vi "Target Analyze.vi"(0 "Original Image_in":T1, 1 "Target Choice":i8(knob) scale=0.0..2.0, 5 "Color Plane":i32(ring) items=["Red", "Green", "Blue", "Hue", "Saturation", "Luminance", "Value", "Intensity"], 7 "Range":cluster{"Lower value":sgl, "Upper value":sgl}={"Lower value"=150.0, "Upper value"=255.0} {"Lower value" scale=0.0..255.0; "Upper value" scale=0.0..255.0}, 9 "Camera Type":enum16{"206", "1011"}(ring)=enum."1011", 11 "Annotate":bool=TRUE) -> (3 "Target Info":T2(array[cluster]), 4 "Original Image_out":T1(plugin-control), 6 "Processed Image":T1(plugin-control), 8 "Distance [m]":dbl, 10 "Position of Target Center X":dbl, 14 "Center Target":bool, 15 "Position of Target Center Y":dbl)   [LabVIEW 2012]
doc: "This VI demonstrates how to do target processing on a laptop computer. It uses the same MJPG VI as the dashboard, sets a few of the important camera properties that impact processing, and carries out the same processing steps as the RT example also included in this project."
uses:
  <vilib>/vision/Image Controls.llb/IMAQ Image.ctl
  <vilib>/vision/NI_Vision_Development_Module.lvlib
panel:
  out "Target":bool
  out "Numeric Target Info (X,Y,D)":dbl[](array[numeric])
  in  "Area Size Limit %":dbl=0.5
  in  "Particle Count Limit":i32=10
  in  "Score Limits":T3={"Rect Coverage"=60.0, "X Edge Strength"=40.0, "Y Edge Strength"=60.0, "Center"=75.0, "Outer"=75.0}
  in  "Processing":enum32{"Monochrome", "Color"}(tab)
  out "Value 2":cluster{i32, i32}
  out "Saturation 2":cluster{i32, i32}
  in  "Value":i32=255
  in  "Saturation":i32=255
  in  "Hue 2":i32(knob)=65 scale=0.0..255.0
  in  "Margins":cluster{"Hue":i32, "Sat":i32, "Val":i32}={"Hue"=33, "Sat"=53, "Val"=9} {"Sat" scale=0.0..80.0; "Val" scale=0.0..80.0; "Hue" scale=0.0..80.0}
  out "Hue":cluster{i32, i32}
  # "Information:\nProcessing can be based on color or light intensity.\nParticles within the image are scored by rectangle coverage, aspect ratio, and\nedge strength/hollowness. A particle is considered a target if all scores\nare above the score limits you set. Particles can be annotated -- surrounded by\na rectangle and scores drawn to the left .\nTo control the number of particles being scored, use the count limit and the size\nlimit.\nBe sure to set the Camera IP before running. The distance calculation uses the\ncamera type to index the value of the lens view angle."
  # "Click in the image to choose  color for processing."
  # "Green scores are above the limit, orange are below. Inner/outer rect\nindicates all passed."
  # "Lower/Upper"
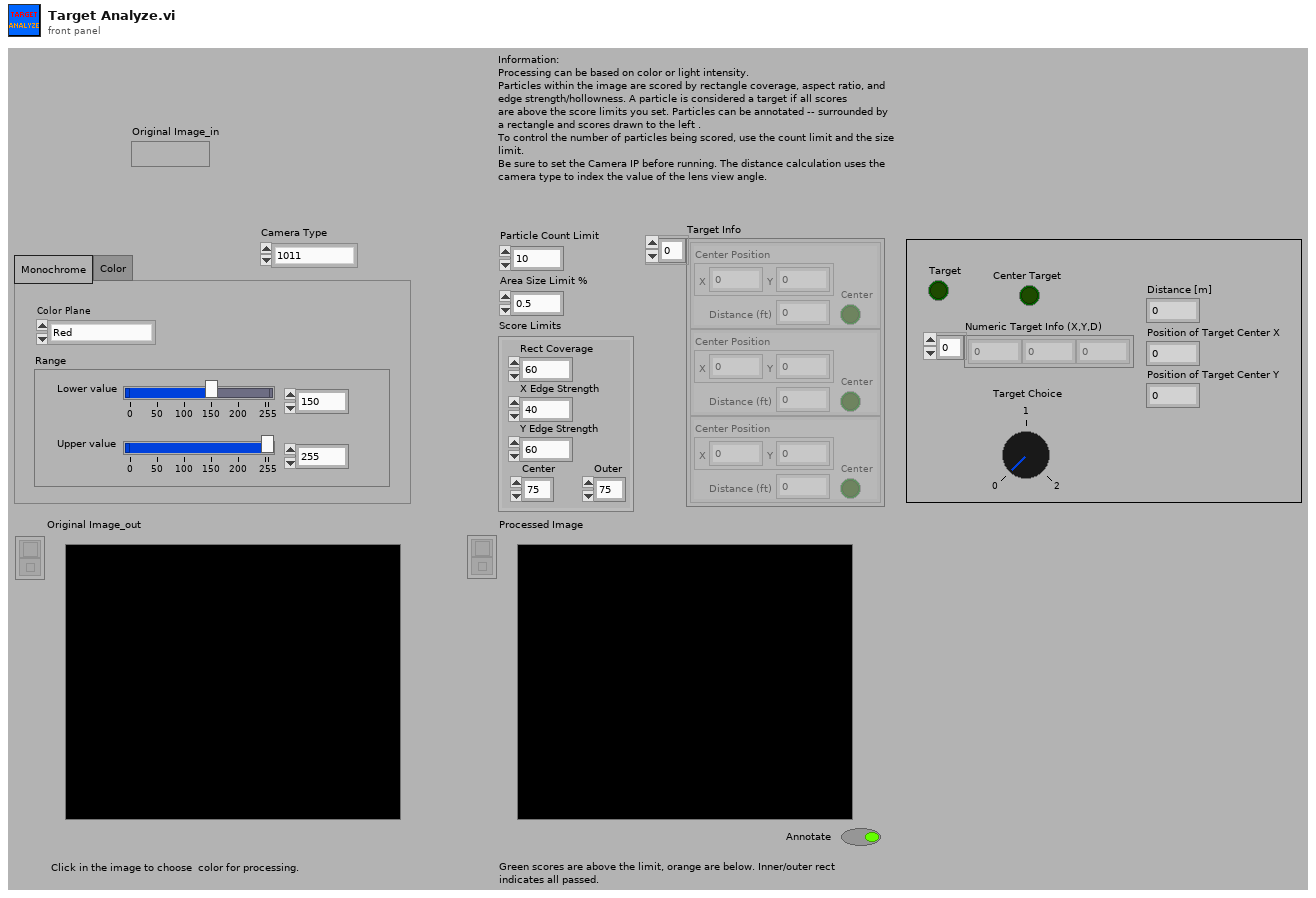
[diagram p1: front panel]
types:
  T1 = typedef "IMAQ Image.ctl" = refnum<image>
  T2 = cluster{"Center Position":cluster{"X":dbl, "Y":dbl}, "Distance (ft)":dbl, "Center":bool}[]
  T3 = cluster{"Rect Coverage":dbl, "X Edge Strength":dbl, "Y Edge Strength":dbl, "Center":dbl, "Outer":dbl}
  T4 = cluster{"Position":cluster{"X":dbl, "Y":dbl}, "Distance (ft)":dbl, "Center Target":bool}[]
  T5 = typedef "Image Type" = u32
  T6 = cluster{cluster{"Left":dbl, "Top":dbl, "Right":dbl, "Bottom":dbl}, "Scores":dbl[], cluster{"Long":dbl, "Short":dbl}}[]
  T7 = cluster{"Target Center (-1 to 1)":cluster{"X":dbl, "Y":dbl}, "Distance (ft)":dbl, "Center Target":bool}
  T8 = cluster{"Target Center (-1 to 1)":cluster{"X":dbl, "Y":dbl}, "Distance (ft)":dbl, "Center Target":bool}[]
  T9 = cluster{"Position":cluster{"X":dbl, "Y":dbl}, "Distance (ft)":dbl, "Center Target":bool}
  T10 = cluster{"Left":dbl, "Top":dbl, "Right":dbl, "Bottom":dbl}
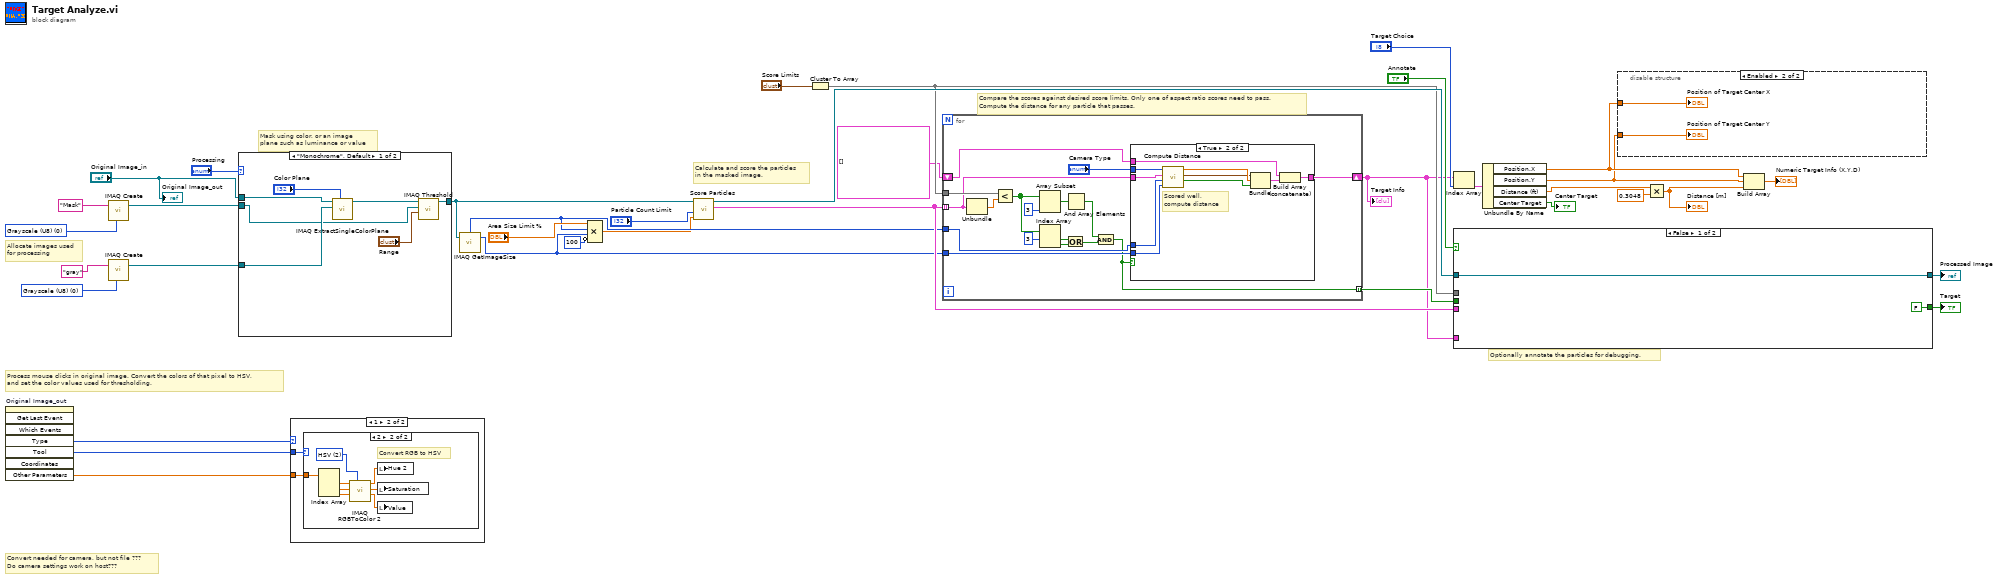
[diagram p0: block diagram]
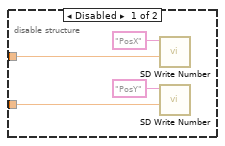
[diagram p2: hidden frame]
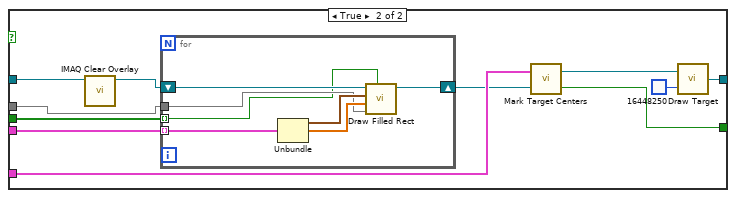
[diagram p3: hidden frame]
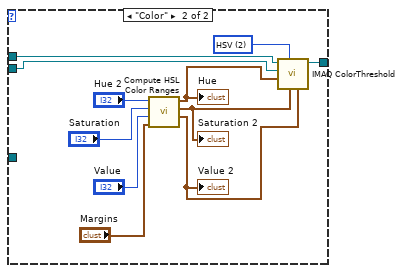
[diagram p4: hidden frame]
diagram:
  w33 = T5 0 items=["Grayscale (U8)", "Grayscale (I16)", "Grayscale (SGL)", "Complex (CSG)", "RGB (U32)", "HSL (U32)", "RGB (U64)", "Grayscale (U16)"] ("Image Type")
  w37 = T5 0 items=["Grayscale (U8)", "Grayscale (I16)", "Grayscale (SGL)", "Complex (CSG)", "RGB (U32)", "HSL (U32)", "RGB (U64)", "Grayscale (U16)"] ("Image Type")
  # "Optionally annotate the particles for debugging."
  # "Compare the scores against desired score limits. Only one of aspect ratio scores need to pass.\nCompute the distance for any particle that passes."
  # "Process mouse clicks in original image. Convert the colors of that pixel to HSV,\nand set the color values used for thresholding."
  # "Calculate and score the particles\nin the masked image."
  # "Mask using color, or an image\nplane such as luminance or value"
  # "Convert needed for camera, but not file ???\nDo camera settings work on host???"
  # "Allocate images used\nfor processing"
  n1 = invoke on="Original Image_out" class="ImageControl" method="Get Last Event"() -> ("Type"=w28:i32, "Tool"=w29:i32, "Other Parameters"=w30:sgl[])  [unwired: 8 in, 5 out]
  n2 = call "IMAQ Create"("Image Name"="Mask", "Image Type"=w33) -> ("New Image"=w32:T1)  [unwired: 2 in, 2 out]
  n3 = call "IMAQ Create"("Image Name"="gray", "Image Type"=w37) -> ("New Image"=w35:T1)  [unwired: 2 in, 2 out]
  n4 = case shown="\"Monochrome\", Default" "Processing" {
    tunnel: "Original Image_in" -> [w44 w55]
    tunnel: w35 -> [w43 _]
    tunnel: [w40 w54] -> w22
    tunnel: w32 -> [w38 w45]
    frame "Monochrome", Default {
      n5 = call "IMAQ ExtractSingleColorPlane"("Color Plane"="Color Plane", "Image Dst"=w43, "Image Src"=w44) -> ("Image Dst Out"=w42:T1)  [unwired: 1 in, 7 out]
      n6 = call "IMAQ Threshold"("Range"="Range", "Image Dst"=w38, "Image Src"=w42) -> ("Image Dst Out"=w40:T1)  [unwired: 3 in, 5 out]
    }
    frame "Color" {
      w53 = u16 2 items=["RGB", "HSL", "HSV", "HSI"] ("Color Mode")
      n7 = call "Compute HSL Color Ranges.vi"("Margins"="Margins", "Luminance"="Value", "Saturation"="Saturation", "Hue"="Hue 2") -> ("Lum Range"=w46:cluster{i32, i32}, "Sat Range"=w47:cluster{i32, i32}, "Hue Range"=w52:cluster{i32, i32})  [unwired: 5 in]
      "Hue" <- w52
      "Saturation 2" <- w47
      "Value 2" <- w46
      n8 = call "IMAQ ColorThreshold"("Blue or Luma or Val or Inten Range"=w46, "Green or Sat Range"=w47, "Color Mode"=w53, "Red or Hue Range"=w52, "Image Dst"=w45, "Image Src"=w55) -> ("Image Dst Out"=w54:T1)  [unwired: 4 in, 1 out]
    }
  }
  n9 = case shown="1" w28 {
    tunnel: w29 -> [_ w57]
    tunnel: w30 -> [_ w56]
    frame 0, Default {
    }
    frame 1 {
      n10 = case shown="2" w57 {
        tunnel: w56 -> [_ w65]
        frame Default {
        }
        frame 2 {
          w64 = u16 2 items=["RGB", "HSL", "HSV", "HSI", "CIE L*a*b*", "CIE XYZ"] ("Color Mode")
          # "Convert RGB to HSV"
          n11 = Index Array(array=w65) -> (element #1=w63:sgl, element #2=w61:sgl, element #3=w59:sgl)  [unwired: 3 in]
          n12 = call "IMAQ RGBToColor 2"("Color Mode"=w64, "Blue value"=w59, "Green value"=w61, "Red value"=w63) -> ("Blue or Luma or Val or Inten or Z or b*value"=w58:dbl, "Green or Sat or Y or a* value"=w60:dbl, "Red or Hue or X or L* value"=w62:dbl)  [unwired: 4 in, 1 out]
          n13 = local write "Hue 2"(w62) -> ()
          n14 = local write "Saturation"(w60) -> ()
          n15 = local write "Value"(w58) -> ()
        }
      }
    }
  }
  n16 = call "IMAQ GetImageSize"("Image"=w22) -> ("Y Resolution"=w16:i32, "X Resolution"=w17:i32)  [unwired: 3 in, 1 out]
  n17 = Compound Arithmetic op=MULTIPLY("Area Size Limit %", w17, w16, invert 100 ("value")) -> (w15:dbl)
  n18 = call "Score Particles.vi"("Area Size Limit"=w15, "Particle Count Limit"="Particle Count Limit", "Image Refnum in"=w22) -> ("Scored Particle Info"=w24:T6, "Image Refnum out"=w27:T1)  [unwired: 7 in]
  n19 = Cluster To Array(cluster="Score Limits") -> (array=w20:dbl[])
  n20 = for {
    shift-right: [w81] -> w2
    shift-left: T4 [] -> [w82]
    tunnel: w17 -> [w80]
    tunnel: w24 -> [w66] mode=indexing
    tunnel: w20 -> [w78]
    tunnel: w16 -> [w77]
    tunnel: [w68] -> w19 mode=indexing
    n21 = Unbundle(w66) -> ("Scores"=w79:dbl[])  [unwired: 2 out]
    n22 = Less?(x=w78, y=w79) -> (x < y?=w74:bool[])
    n23 = Array Subset(array=w74, length=3) -> (w75:bool[])  [unwired: 1 in]
    n24 = Index Array(array=w74, index #1=3 ("length")) -> (element #1=w72:bool, element #2=w71:bool)  [unwired: 1 in]
    n25 = Or(x=w72, y=w71) -> (x .or. y?=w70:bool)
    n26 = And Array Elements(Boolean array=w75) -> (logical AND=w69:bool)
    n27 = And(x=w69, y=w70) -> (x .and. y?=w68:bool)
    n28 = case shown="True" w68 {
      tunnel: w82 -> [w83 w93]
      tunnel: [w83 w92] -> w81
      tunnel: w80 -> [_ w91]
      tunnel: "Camera Type" -> [_ w89]
      tunnel: w77 -> [_ w87]
      tunnel: w66 -> [_ w86]
      frame False {
        # "Didn't score well enough"
      }
      frame True {
        # "Scored well,\ncompute distance"
        n29 = call "Compute Distance.vi"("Y Image Resolution"=w87, "X Image Resolution"=w91, "Particle Scores"=w86, "Camera Type"=w89) -> ("Center Target"=w85:bool, "Target Center (-1 to 1)"=w88:cluster{"X":dbl, "Y":dbl}, "Distance (ft)"=w90:dbl)  [unwired: 5 in]
        n30 = Bundle("Target Center (-1 to 1)"=w88, "Distance (ft)"=w90, "Center Target"=w85) -> (w84:T7)  [unwired: 1 in]
        n31 = Build Array (concatenate)(w93, w84) -> (w92:T8)
      }
    }
  }
  "Target Info" <- w2
  n32 = Index Array(array=w2, index="Target Choice") -> (element=w10:T9)
  n33 = case shown="False" "Annotate" {
    tunnel: w27 -> [w95 w106]
    tunnel: [w95 w100] -> w25
    tunnel: w24 -> [_ w102]
    tunnel: w20 -> [_ w104]
    tunnel: w19 -> [_ w103]
    tunnel: w2 -> [_ w99]
    tunnel: [FALSE ("Target") w96] -> w1
    frame False {
    }
    frame True {
      n34 = call "IMAQ Clear Overlay"("Image"=w106) -> ("Image Out"=w105:T1)  [unwired: 2 in, 8 out]
      n35 = for {
        shift-right: [w107] -> w98
        shift-left: w105 -> [w113]
        tunnel: w102 -> [w110] mode=indexing
        tunnel: w104 -> [w109]
        tunnel: w103 -> [w108] mode=indexing
        n36 = Unbundle(w110) -> (w111:T10, "Scores"=w112:dbl[])  [unwired: 1 out]
        n37 = call "Draw Filled Rect.vi"("Limit Passed"=w108, "Limits"=w109, "Scores"=w112, "Bounding Box"=w111, "image in"=w113) -> ("image out"=w107:T1)  [unwired: 6 in]
      }
      n38 = call "Mark Target Centers.vi"("Processed Image"=w98, "Target Info"=w99) -> ("Target"=w96:bool, "Image Out"=w97:T1)
      n39 = call "Draw Target.vi"("Color"=u32 16448250, "Original Image"=w97) -> ("Image Out"=w100:T1)
    }
  }
  "Processed Image" <- w25
  "Target" <- w1
  n40 = Unbundle By Name(w10) -> ("Position.X"=w7:dbl, "Position.Y"=w6:dbl, "Distance (ft)"=w8:dbl, "Center Target"=→"Center Target":bool)
  n41 = disable-structure shown="Enabled" {
    disable-tunnel: w7 -> [w115 w119]
    disable-tunnel: w6 -> [w114 w118]
    frame Disabled {
      n42 = call <vilib>:"SD Write Number.vi"("Numeric"=w115, "Name"="PosX") -> ()  [unwired: 8 in, 2 out]
      n43 = call <vilib>:"SD Write Number.vi"("Numeric"=w114, "Name"="PosY") -> ()  [unwired: 8 in, 2 out]
    }
    frame Enabled {
      "Position of Target Center X" <- w119
      "Position of Target Center Y" <- w118
    }
  }
  n44 = Multiply(x=w8, y=0.3048) -> (x*y=w5:dbl)
  "Distance [m]" <- w5
  n45 = Build Array(w7, w6, w5) -> (→"Numeric Target Info (X,Y,D)":dbl[])
  "Original Image_out" <- "Original Image_in"
